vi "Write Global Locked.vi"(8 "error in (no error)":errorcluster, 10 "Global":refnum<class "System.lvclass">, 11 "GrabberArms in":refnum<class "GrabberArms.lvclass">) -> (0 "error out":errorcluster, 3 "GrabberArms out":refnum<class "GrabberArms.lvclass">)   [LabVIEW 2013, in "GrabberArms.lvclass"]
uses:
  GrabberArms.lvclass
  System/System.lvclass
  Robot Global Data.vi
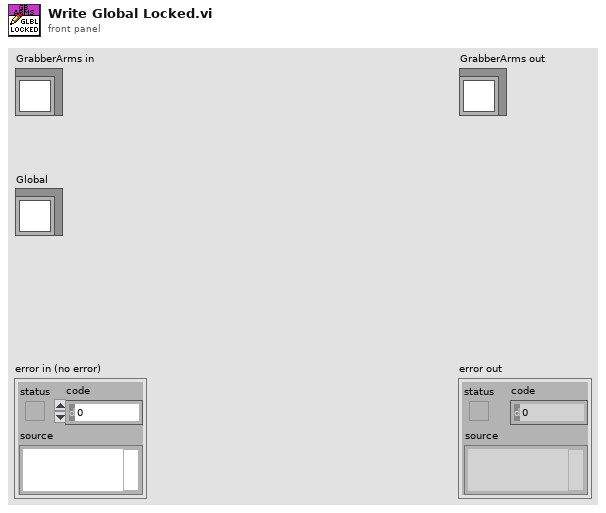
[diagram p1: front panel]
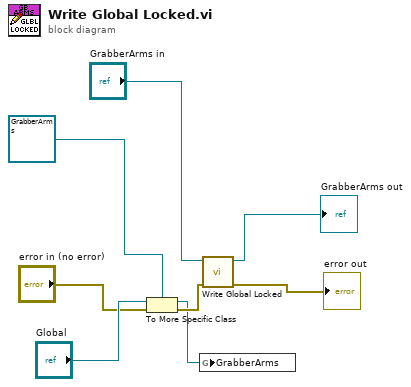
[diagram p0: block diagram]
diagram:
  n1 = To More Specific Class(target class=refnum<class "GrabberArms.lvclass"> refnum ("GrabberArms.lvclass"), reference="Global", error in="error in (no error)") -> (specific class reference=w2:refnum<class "GrabberArms.lvclass">, error out=w3:errorcluster)
  n2 = global write "Robot Global Data.vi" "GrabberArms"(w2) -> ()
  n3 = call-parent "Write Global Locked.vi"("error in (no error)"=w3, "System in"="GrabberArms in") -> ("error out"=→"error out":errorcluster, "System out"=→"GrabberArms out":refnum<class "GrabberArms.lvclass">)  [unwired: 8 in]
